vi "Initial Values-format and values-STRING.vi"() -> (1 "Values Array":string[](array[string]), 3 "Keys Array":T1)   [LabVIEW 2013]
uses:
  Typedefs/Ini file interface (String).ctl
  Global Variables/gl_UI Ctrl Refs.vi
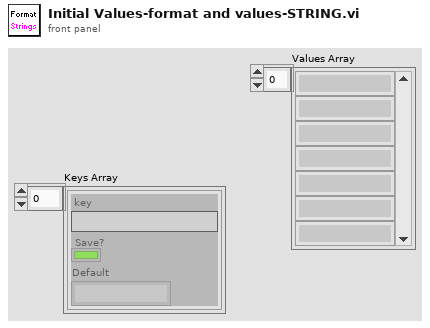
[diagram p1: front panel]
types:
  T1 = typedef "Ini file interface (String).ctl" = cluster{"key":string, "Save?":bool, "Default":string}[]
  T2 = cluster{"key":string, "Save?":bool, "Default":string}
  T3 = typedef "UI ctrl refs cluster.ctl" = cluster{"Top level VI path":path, "Top level VI ref":refnum<vi>, "User menu ref":refnum<k9>, "Sub Panel control":refnum<vi>, "Imaging Param Tab":refnum<vi>, "Occurrence-Start drivers":refnum<k4>, "Occurrence-Speed logging initialised":refnum<k4>, "Occurrence-XYZ stage initialised":refnum<k4>, "Exit button":refnum<vi>, "Status ind":refnum<vi>, "Return to Origin":refnum<vi>, "Speed Logging":refnum<vi>, "Time Lapse":refnum<vi>, "Live Imaging":refnum<vi>, "AOL Z Stack":refnum<vi>, "Motor Z Stack":refnum<vi>, "Funct Acq button":refnum<vi>, "Hard Shutter":refnum<vi>, "Virtual Shutter":refnum<vi>, "Laser Power":refnum<vi>, "AOL Mode":refnum<vi>, "Frame Size":refnum<vi>, "Field of View":refnum<vi>, "Dwell Time":refnum<vi>, "Zoom":refnum<vi>, "AOL Z":refnum<vi>, "Objective":refnum<vi>, "Axis":refnum<vi>, "Paths & Names":refnum<vi>, "Experiment folder path (ind.)":refnum<vi>, "Last State (Ind.)":refnum<vi>, "Laser wavelength ind (nm)":refnum<vi>, "Averages":refnum<vi>, "Angle (degrees)":refnum<vi>, "X centre":refnum<vi>, "Y centre":refnum<vi>, "Plane Mode":refnum<vi>, "# Planes":refnum<vi>, "Z Start":refnum<vi>, "Z Stop":refnum<vi>, "Z Step":refnum<vi>, "PMT 1":refnum<vi>, "PMT 2":refnum<vi>, "Stage XYZ Position":refnum<vi>, "Pockels@Z Start":refnum<vi>, "Pockels@Z Stop":refnum<vi>, "Obtain Z Start":refnum<vi>, "Obtain Z Stop":refnum<vi>, "Live stim.trig.period":refnum<vi>, "Live stim.trig.enable":refnum<vi>, "Funct. Acq. Pockels Modulation":refnum<vi>, "Enable Video Recording":refnum<vi>, "Video Record-Live Imaging":refnum<vi>, "Video Record-Funct acq":refnum<vi>, "AOL Z-stack Chirps Ready (ind)":refnum<vi>, "Center freq ind (nm)":refnum<vi>, "Logging queue (ind)":refnum<vi>, "Back aperture power (ind.)":refnum<vi>, "Power after objective (ind.)":refnum<vi>, "Switch user":refnum<vi>}
  T4 = cluster{"Base Directory":path, "User folder?":bool, "Sub-Folder":string, "Experiment folder custom name":string}
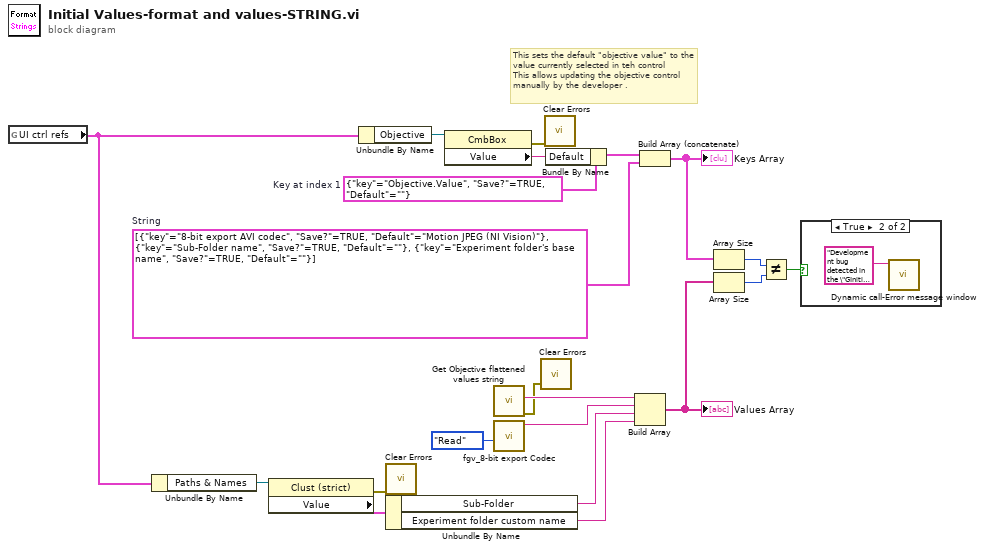
[diagram p0: block diagram]
diagram:
  w18 = T2 {"key"="Objective.Value", "Save?"=TRUE, "Default"=""}  # Key at index 1
  w19 = T1 [{"key"="8-bit export AVI codec", "Save?"=TRUE, "Default"="Motion JPEG (NI Vision)"}, {"key"="Sub-Folder name", "Save?"=TRUE, "Default"=""}, {"key"="Experiment folder's base name", "Save?"=TRUE, "Default"=""}]  # String
  # "This sets the default \"objective value\" to the value currently selected in teh control\nThis allows updating the objective control manually by the developer ."
  n1 = global read "gl_UI Ctrl Refs.vi" "UI ctrl refs"() -> (w3:T3)
  n2 = Unbundle By Name(w3) -> ("Paths & Names"=w5:refnum<vi>)
  n3 = property on="Property Node" class="Clust (strict)"(reference=w5) -> (error out=w6:errorcluster, "Value"=w4:T4)  [unwired: 1 in, 1 out]
  n4 = Unbundle By Name(w3) -> ("Objective"=w16:refnum<vi>)
  n5 = call <vilib>:"Clear Errors.vi"("error in (no error)"=w6) -> ()  [unwired: 6 in, 1 out]
  n6 = Unbundle By Name(w4) -> ("Sub-Folder"=w2:string, "Experiment folder custom name"=w1:string)
  n7 = property on="Property Node" class="CmbBox"(reference=w16) -> (error out=w8:errorcluster, "Value"=w17:string)  [unwired: 1 in, 1 out]
  n8 = call "Get Objective flattened values string.vi"() -> ("error out"=w7:errorcluster, "Objective.Value"=w21:string)  [unwired: 9 in, 1 out]
  n9 = call "fgv_8-bit export Codec.vi"("Function"=enum16{"Intialize", "Write", "Read", "Clear"}."Read") -> ("AVI mode"=w14:string)  [unwired: 9 in, 1 out]
  n10 = call <vilib>:"Clear Errors.vi"("error in (no error)"=w7) -> ()  [unwired: 6 in, 1 out]
  n11 = call <vilib>:"Clear Errors.vi"("error in (no error)"=w8) -> ()  [unwired: 6 in, 1 out]
  n12 = Bundle By Name(cluster=w18, "Default"=w17) -> (w20:T2)
  n13 = Build Array(w21, w14, w2, w1) -> (w10:string[])
  "Values Array" <- w10
  n14 = Build Array (concatenate)(w20, w19) -> (w11:T1)
  "Keys Array" <- w11
  n15 = Array Size(array=w11) -> (size(s)=w13:i32)
  n16 = Array Size(array=w10) -> (size(s)=w12:i32)
  n17 = Not Equal?(x=w13, y=w12) -> (x != y?=w9:bool)
  n18 = case shown="True" w9 {
    frame False {
    }
    frame True {
      n19 = call "Dynamic call-Error message window.vi"("Error Message"="Development bug detected in the \"GInitial Values-format and values-STRING.vi\"") -> ()  [unwired: 10 in, 1 out]
    }
  }
